vi "Get or confirm IP address.vi"(8 "error in":errorcluster) -> (0 "error out":errorcluster)   [LabVIEW 2024, in "Session Scanner.lvlib"]
doc: "Retrieves IP address or Hostname from input data in case the user only knows one of these fields"
uses:
  Session Scanner.lvlib
  <vilib>/Utility/error.llb/Trim Whitespace One-Sided.vi
  Support/General Type Defs/Global Data.vi
  Support/General Type Defs/General Type Defs.lvlib
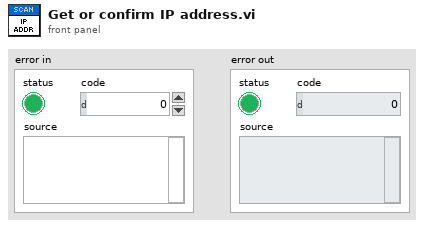
[diagram p1: front panel]
types:
  T1 = typedef "General Type Defs.lvlib/Device Data.ctl" = cluster{"OS":T2, "User":string, "Password":string, "Hostname":string, "IP Address":string}
  T2 = typedef "General Type Defs.lvlib/Device OS.ctl" = enum16{"Windows", "Linux"}
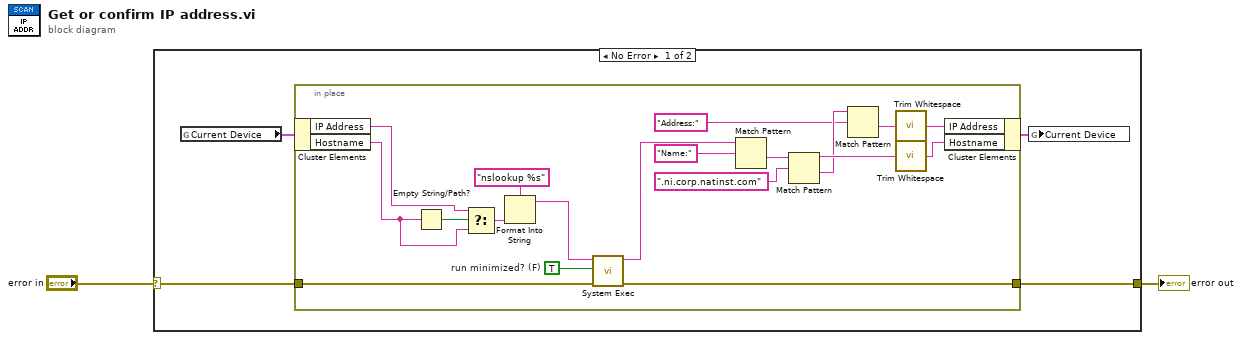
[diagram p0: block diagram]
diagram:
  n1 = case shown="No Error" "error in" {
    selector: "error in" -> [w5 w26]
    tunnel: [w6 w26] -> w2
    frame No Error {
      n2 = global read "Global Data.vi" "Current Device"() -> (w4:T1)
      n3 = in-place {
        in-place-border: [w24] -> w6
        in-place-border: w5 -> [w11]
        w13 = TRUE  # run minimized? (F)
        n4 = in-place-cluster #1(w4) -> ("IP Address"=w10:string, "Hostname"=w9:string)
        n5 = Empty String/Path?(string/path=w9) -> (empty?=w25:bool)
        n6 = Select(t=w10, s=w25, f=w9) -> (s? t:f=w12:string)
        n7 = Format Into String(format string="nslookup %s", w12) -> (resulting string=w18:string)  [unwired: 2 in, 1 out]
        n8 = call <vilib>:"System Exec.vi"("run minimized? (F)"=w13, "error in (no error)"=w11, "command line"=w18) -> ("error out"=w24:errorcluster, "standard output"=w21:string)  [unwired: 5 in, 2 out]
        n9 = Match Pattern(string=w21, regular expression="Name:") -> (after substring=w22:string)  [unwired: 1 in, 3 out]
        n10 = Match Pattern(string=w22, regular expression=".ni.corp.natinst.com") -> (before substring=w23:string, after substring=w19:string)  [unwired: 1 in, 2 out]
        n11 = Match Pattern(string=w19, regular expression="Address:") -> (after substring=w20:string)  [unwired: 1 in, 3 out]
        n12 = call <vilib>:"Trim Whitespace.vi"("string"=w20) -> ("trimmed string"=w7:string)  [unwired: 1 in]
        n13 = call <vilib>:"Trim Whitespace.vi"("string"=w23) -> ("trimmed string"=w8:string)  [unwired: 1 in]
        n14 = in-place-cluster #1("IP Address"=w7, "Hostname"=w8) -> (w3:T1)
      }
      n15 = global write "Global Data.vi" "Current Device"(w3) -> ()
    }
    frame Error {
    }
  }
  "error out" <- w2
